vi "OPC_UA_Server.vi"() -> ()   [LabVIEW 2021]
uses:
  <vilib>/OPCUA/controls/NodeId.ctl
  <vilib>/OPCUA/controls/Data Type.ctl
  <vilib>/OPCUA/NI OPC UA Server.lvlib
panel:
  out "item node ID":T1
  in  "stop":bool
  out "server endpoint URL":string
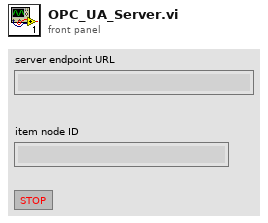
[diagram p1: front panel]
types:
  T1 = typedef "NodeId.ctl" = string
  T2 = typedef "Data Type.ctl" = u16
  T3 = cluster{"name":string, "data type":T2, "access level":u16, "description":string}
  T4 = typedef "OPC UA Server Refnum.ctl" = refnum<k21>
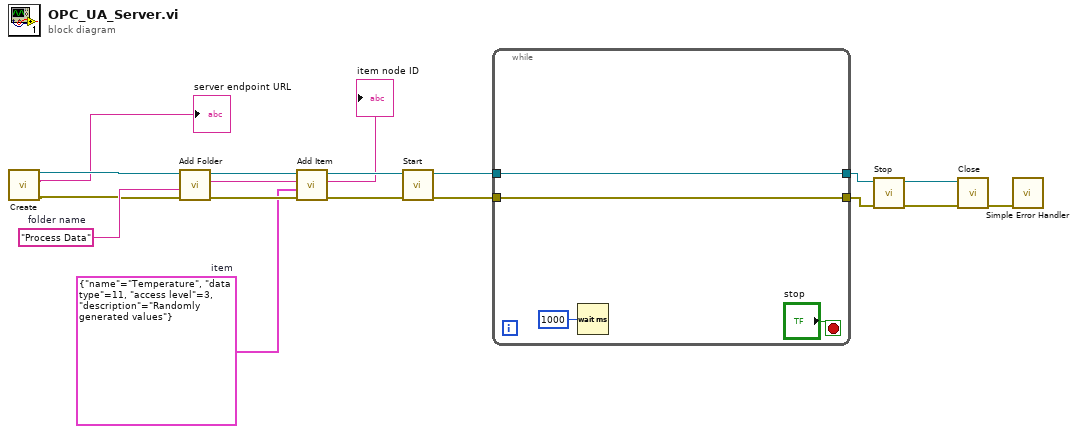
[diagram p0: block diagram]
diagram:
  w6 = T3 {"name"="Temperature", "data type"=11, "access level"=3, "description"="Randomly generated values"}  # item
  w8 = "Process Data"  # folder name
  n1 = call <vilib>:"Create.vi"() -> ("error out"=w1:errorcluster, "server endpoint URL"=→"server endpoint URL":string, "OPC UA server refnum out"=w3:T4)  [unwired: 9 in]
  n2 = call <vilib>:"Add Folder.vi"("error in (no error)"=w1, "folder name"=w8, "OPC UA server refnum in"=w3) -> ("error out"=w13:errorcluster, "folder node ID"=w7:T1, "OPC UA server refnum out"=w18:T4)  [unwired: 5 in]
  n3 = call <vilib>:"Add Item.vi"("error in (no error)"=w13, "item"=w6, "parent folder node ID"=w7, "OPC UA server refnum in"=w18) -> ("error out"=w12:errorcluster, "item node ID"=→"item node ID":T1, "OPC UA server refnum out"=w17:T4)  [unwired: 3 in, 1 out]
  n4 = call <vilib>:"Start.vi"("error in (no error)"=w12, "OPC UA server refnum in"=w17) -> ("error out"=w11:errorcluster, "OPC UA server refnum out"=w16:T4)  [unwired: 7 in, 1 out]
  n5 = while {
    tunnel: w16 -> [w20]
    tunnel: [w20] -> w15
    tunnel: w11 -> [w19]
    tunnel: [w19] -> w10
    stop <- "stop" stop-if-true
    n6 = Wait (ms)(milliseconds to wait=u32 1000) -> ()  [unwired: 1 out]
  }
  n7 = call <vilib>:"Stop.vi"("error in (no error)"=w10, "OPC UA server refnum in"=w15) -> ("error out"=w9:errorcluster, "OPC UA server refnum out"=w14:T4)  [unwired: 8 in]
  n8 = call <vilib>:"Close.vi"("error in (no error)"=w9, "OPC UA server refnum in"=w14) -> ("error out"=w4:errorcluster)  [unwired: 9 in]
  n9 = call <vilib>:"Simple Error Handler.vi"("error in (no error)"=w4) -> ()  [unwired: 4 in, 5 out]
